vi "Write Data.vi"(8 "error in (no error)":errorcluster, 10 "Data":variant, 11 "Tag_LVOOP.lvclass in":refnum<class "Tree Tag Class.lvclass">) -> (0 "error out":errorcluster, 3 "Tag_LVOOP.lvclass out":refnum<class "Tree Tag Class.lvclass">)   [LabVIEW 2012, in "Tree Tools.lvlib" / "Tree Tag Class.lvclass"]
uses:
  Tree Tag Class.lvclass
  Tree Tag Class.lvclass/Tree Tag Class.ctl
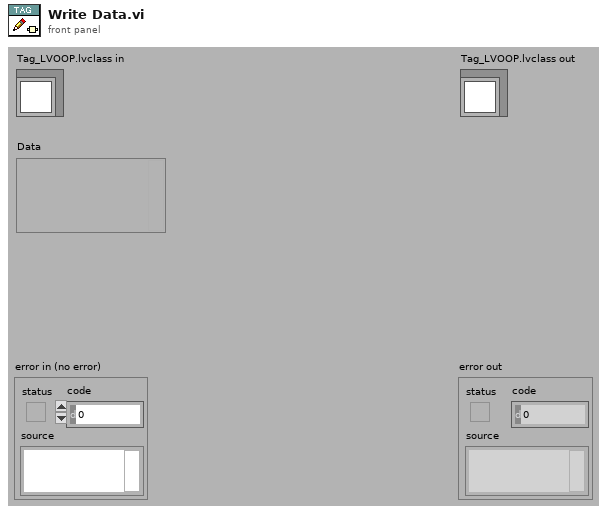
[diagram p1: front panel]
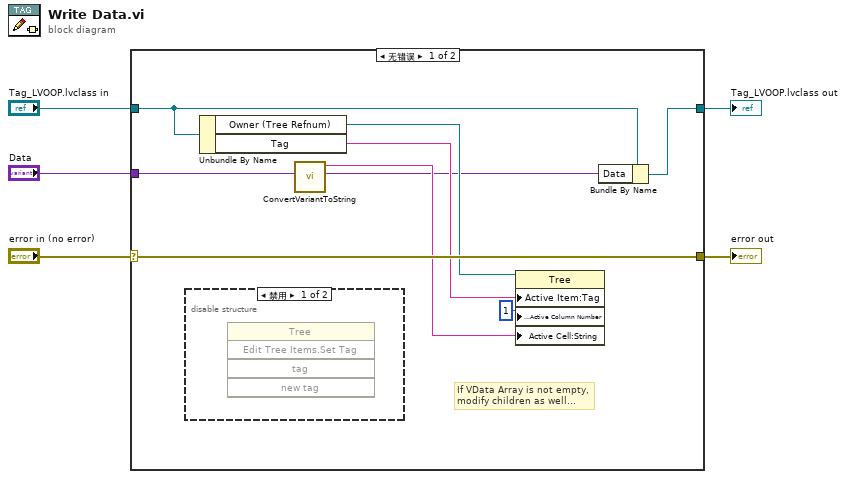
[diagram p0: block diagram]
diagram:
  n1 = case shown="无错误" "error in (no error)" {
    selector: "error in (no error)" -> [w14 w15]
    tunnel: [w14 w15] -> w4
    tunnel: [w13 w16] -> w2
    tunnel: "Tag_LVOOP.lvclass in" -> [w12 w16]
    tunnel: "Data" -> [w7 _]
    frame No Error {
      # "If VData Array is not empty,\nmodify children as well..."
      n2 = disable-structure shown="禁用" {
        frame Disabled {
          n3 = invoke class="Tree" method="Edit Tree Items.Set Tag"() -> ()  [unwired: 5 in, 5 out]
        }
        frame Enabled {
        }
      }
      n4 = Unbundle By Name(w12) -> ("Owner (Tree Refnum)"=w11:refnum<vi>, "Tag"=w10:string)
      n5 = call "ConvertVariantToString.vi"("Variant"=w7) -> ("Variant dup"=w6:variant, "String"=w8:string)  [unwired: 1 in, 8 out]
      n6 = property class="Tree"(reference=w11, "Active Item:Tag"=w10, "Active Cell:Active Column Number"=1, "Active Cell:String"=w8) -> ()  [unwired: 1 in, 2 out]
      n7 = Bundle By Name(cluster=w12, "Data"=w6) -> (w13:refnum<class "Tree Tag Class.lvclass">)
    }
    frame Error {
    }
  }
  "error out" <- w4
  "Tag_LVOOP.lvclass out" <- w2
